vi "AccueilAdministrateur.vi"() -> ()   [LabVIEW 2015]
uses:
  Queues and Variants 8.2/Queue Element.ctl
  Queues and Variants 8.2/Data Type.ctl
  <vilib>/httpClient/LabVIEWHTTPClient.lvlib
panel:
  in  "OK Button 8":bool
  out "Boolean Out":bool
  out "String Out":string
  out "Double Precision Out":dbl
  in  "OK Button 7":bool
  in  "OK Button 6":bool
  in  "OK Button 5":bool
  in  "OK Button 4":bool
  in  "OK Button 3":bool
  in  "OK Button 2":bool
  in  "OK Button":bool
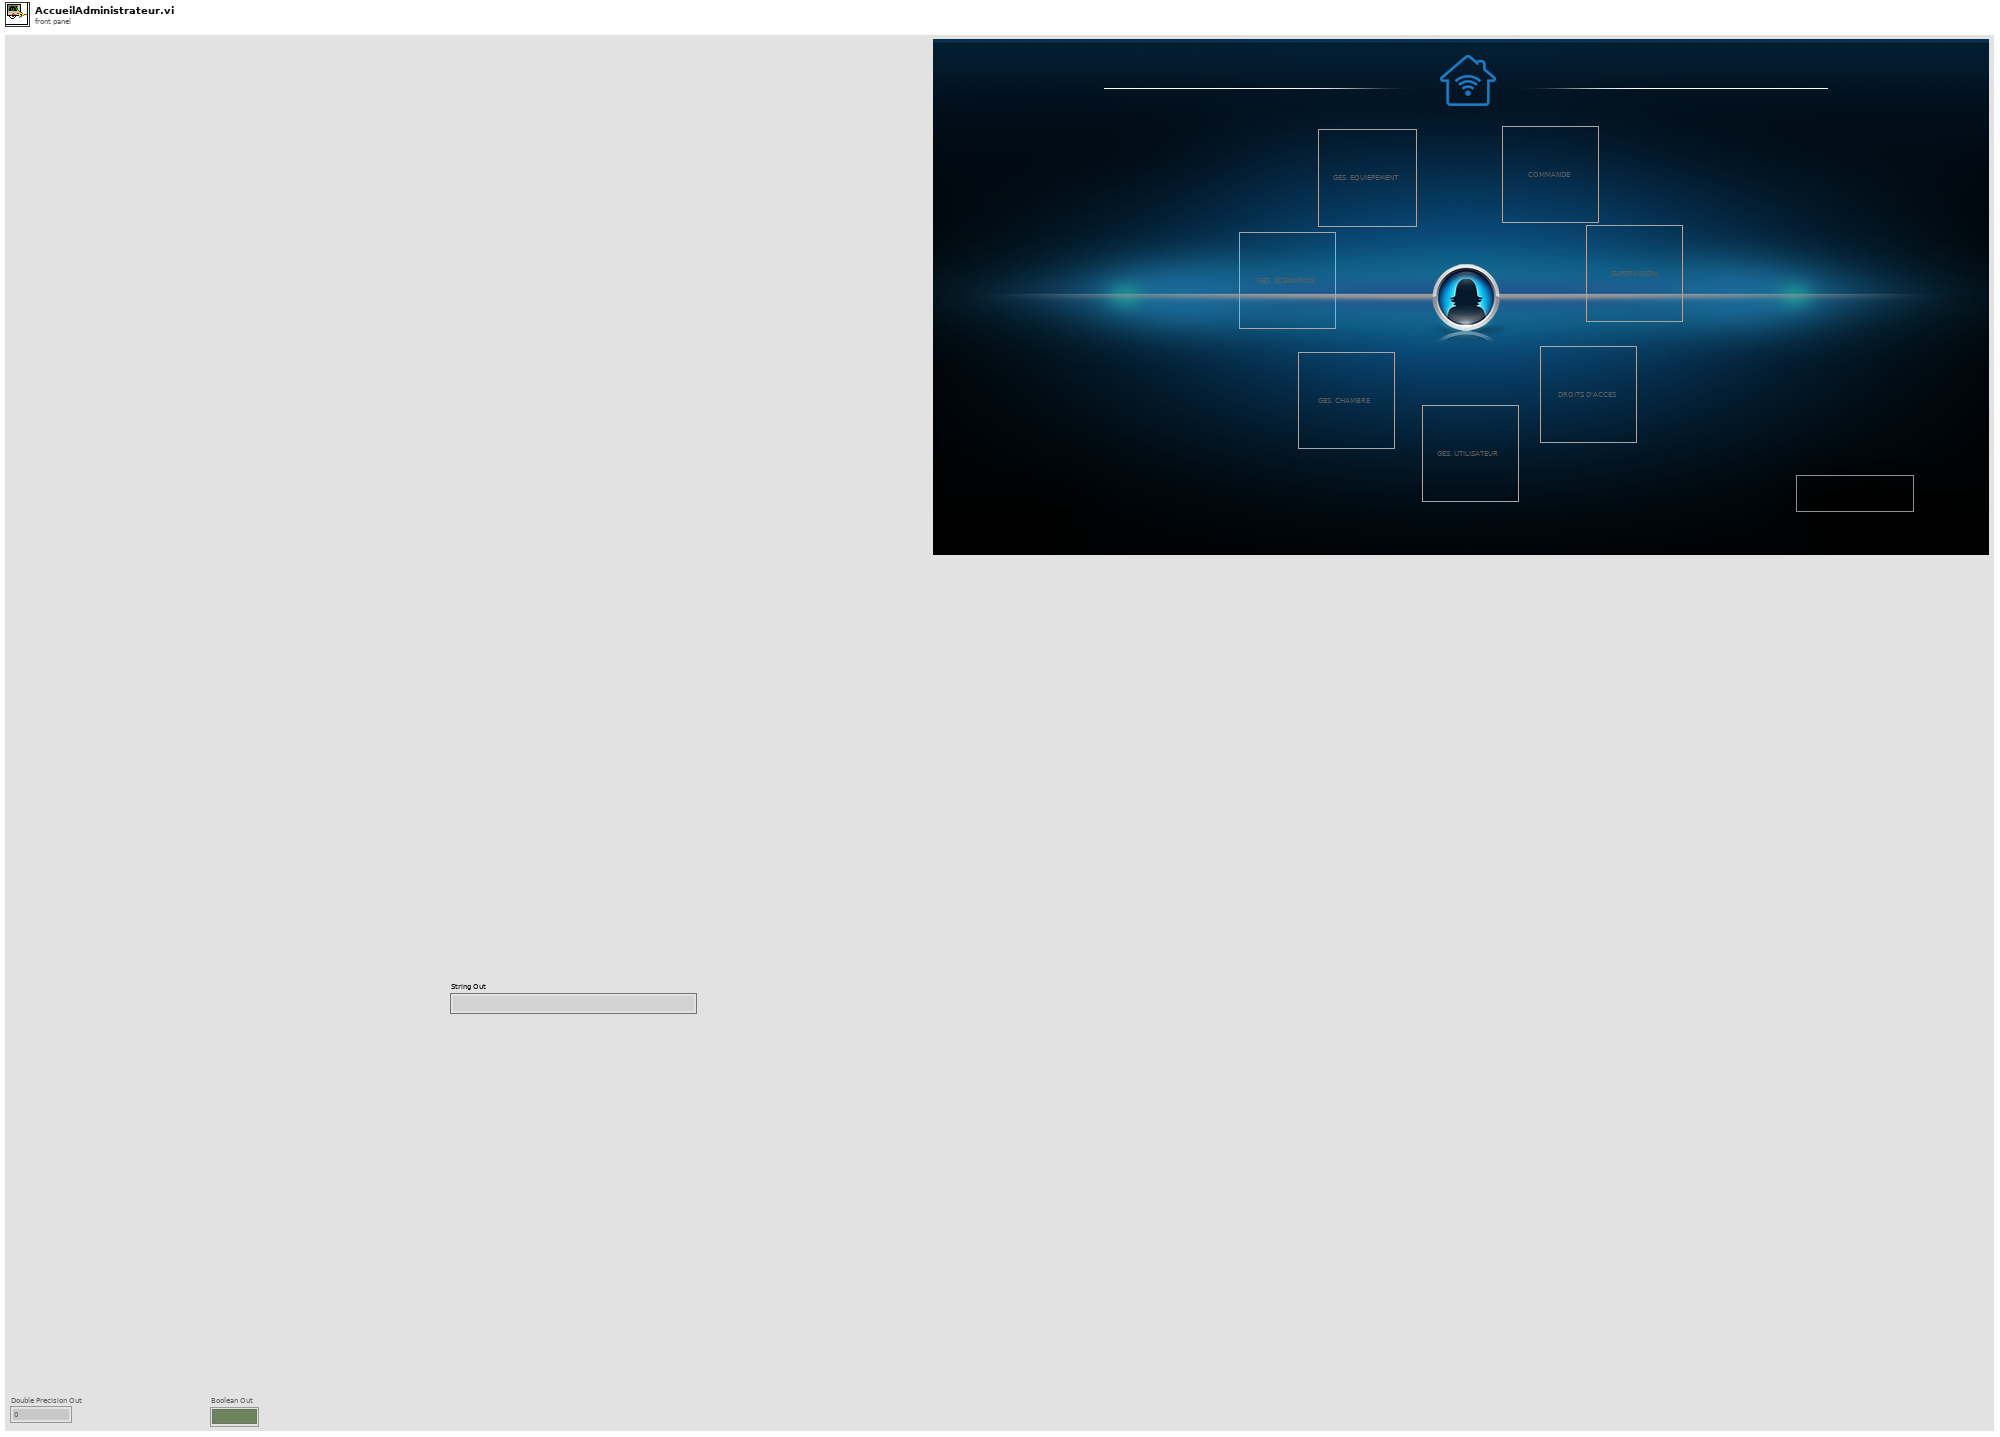
[diagram p1: front panel]
types:
  T1 = typedef "Queue Element.ctl" = cluster{"Data Type":T2, "Variant":variant}
  T2 = typedef "Data Type.ctl" = enum16{"Double Precision", "String", "Boolean"}
  T3 = enum32{"Invalid", "Standard", "Closed", "Hidden", "Minimized", "Maximized"}
  T4 = enum8{"Enabled", "Disabled", "Disabled and Grayed Out"}
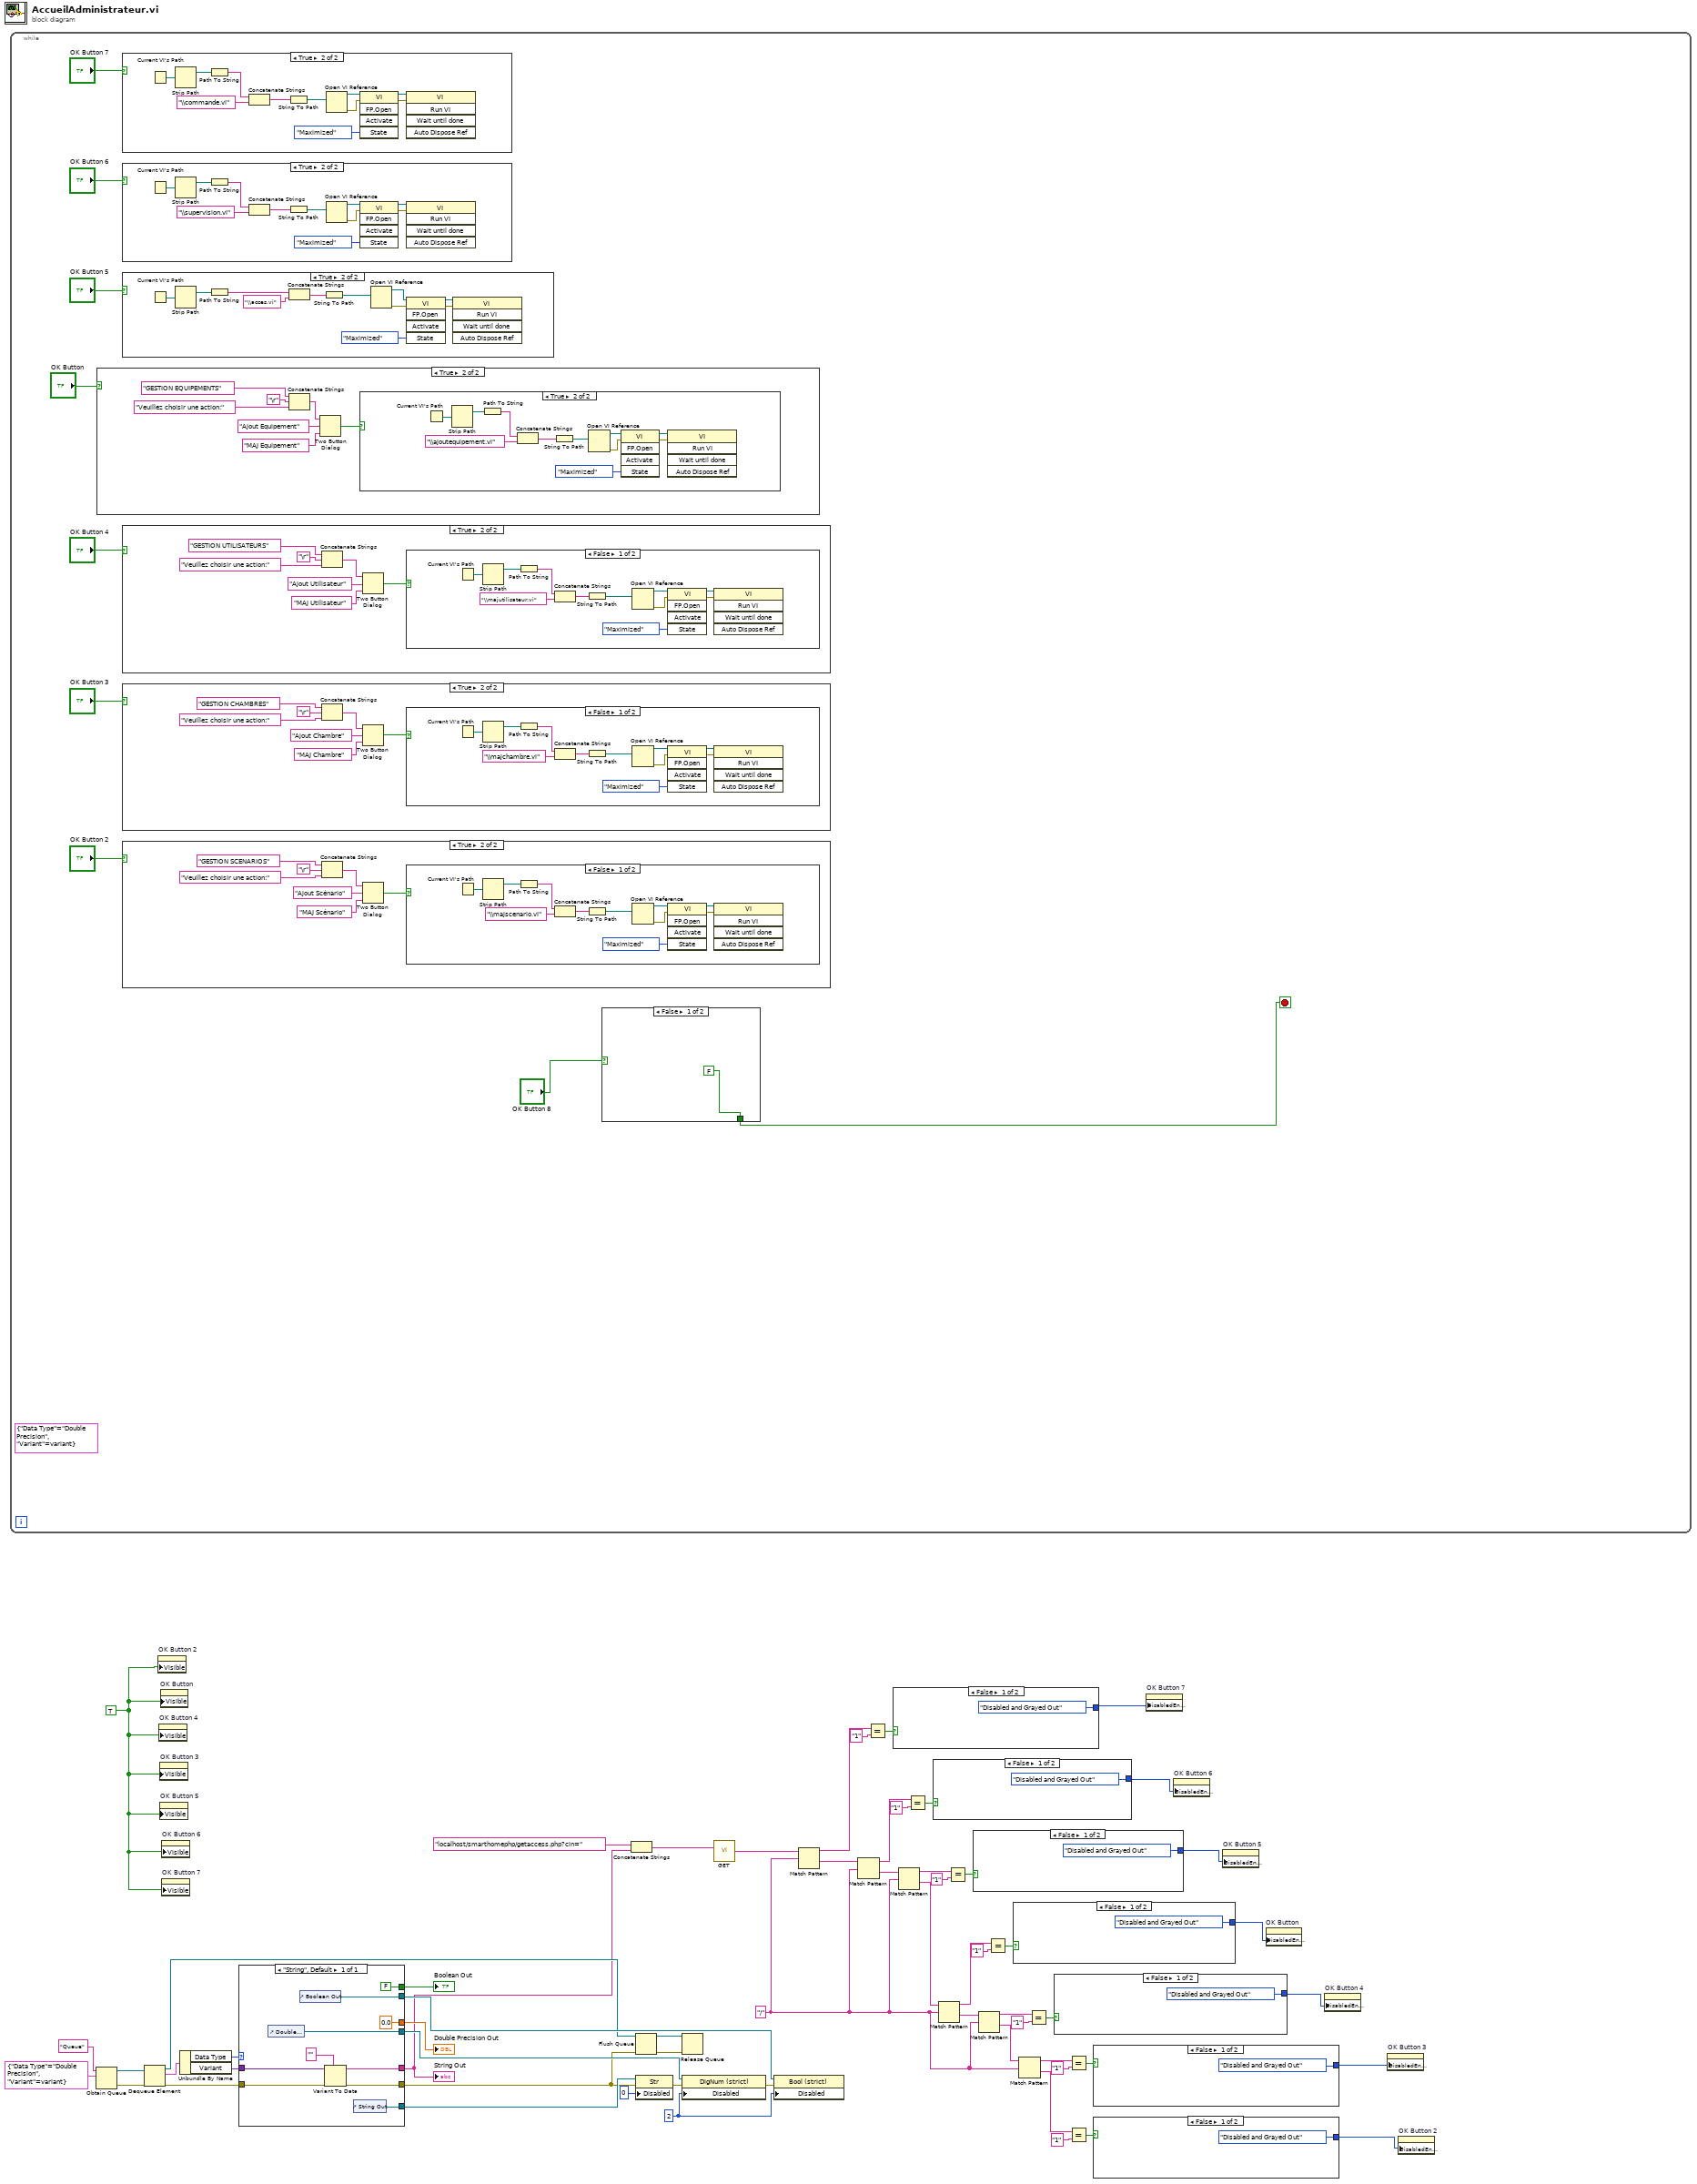
[diagram p0: block diagram]
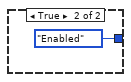
[diagram p2: hidden frame]
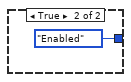
[diagram p3: hidden frame]
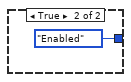
[diagram p4: hidden frame]
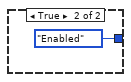
[diagram p5: hidden frame]
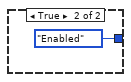
[diagram p6: hidden frame]
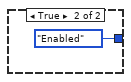
[diagram p7: hidden frame]
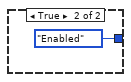
[diagram p8: hidden frame]
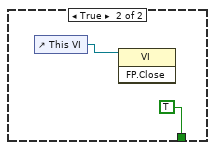
[diagram p9: hidden frame]
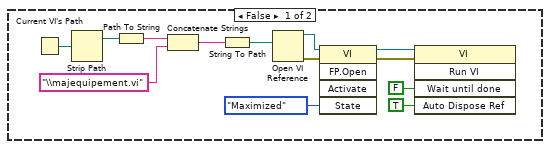
[diagram p14: hidden frame]
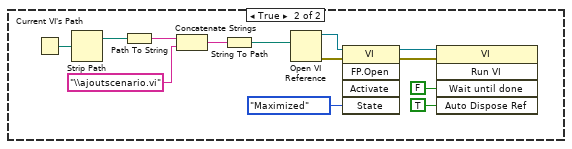
[diagram p16: hidden frame]
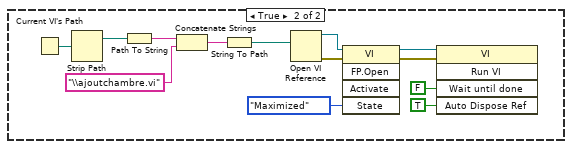
[diagram p18: hidden frame]
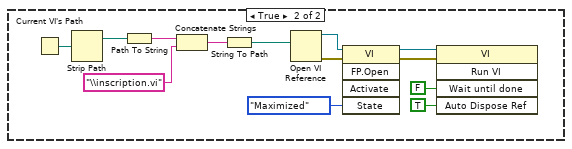
[diagram p20: hidden frame]
diagram:
  w26 = "/" ("regular expression")
  w44 = u8 2 ("Disabled")
  w53 = TRUE
  n1 = while {
    stop <- w61 stop-if-true
    (unwired) T1 {"Data Type"=enum."Double Precision", "Variant"=variant} ("Queue Element")
    n2 = case shown="True" "OK Button" {
      frame False {
      }
      frame True {
        n3 = Concatenate Strings("GESTION EQUIPEMENTS", "\r", "Veuillez choisir une action:" ("message")) -> (w109:string)
        n4 = Two Button Dialog(message=w109, 1:"MAJ Equipement" ("F button name (\"Cancel\")"), 2:"Ajout Equipement" ("T button name (\"OK\")")) -> (T button?=w106:bool)
        n5 = case shown="True" w106 {
          frame False {
            n6 = Current VI's Path() -> (path=w125:path)
            n7 = Strip Path(path=w125) -> (stripped path=w124:path)  [unwired: 1 out]
            n8 = Path To String(path=w124) -> (string=w123:string)
            n9 = Concatenate Strings(w123, "\\majequipement.vi") -> (w121:string)
            n10 = String To Path(string=w121) -> (path=w120:path)
            n11 = Open VI Reference(vi path=w120) -> (vi reference=w119:refnum<vi>, error out=w118:errorcluster)  [unwired: 5 in]
            n12 = invoke class="VI" method="FP.Open"(reference=w119, error in=w118, "State"=T3."Maximized") -> (reference out=w117:refnum<vi>, error out=w116:errorcluster)  [unwired: 2 in, 3 out]
            n13 = invoke class="VI" method="Run VI"(reference=w117, error in=w116, "Wait until done"=FALSE ("Wait Until Done"), "Auto Dispose Ref"=TRUE ("Auto Dispose Reference")) -> ()  [unwired: 1 in, 5 out]
          }
          frame True {
            n14 = Current VI's Path() -> (path=w136:path)
            n15 = Strip Path(path=w136) -> (stripped path=w135:path)  [unwired: 1 out]
            n16 = Path To String(path=w135) -> (string=w134:string)
            n17 = Concatenate Strings(w134, "\\ajoutequipement.vi") -> (w132:string)
            n18 = String To Path(string=w132) -> (path=w131:path)
            n19 = Open VI Reference(vi path=w131) -> (vi reference=w130:refnum<vi>, error out=w129:errorcluster)  [unwired: 5 in]
            n20 = invoke class="VI" method="FP.Open"(reference=w130, error in=w129, "State"=T3."Maximized") -> (reference out=w128:refnum<vi>, error out=w127:errorcluster)  [unwired: 2 in, 3 out]
            n21 = invoke class="VI" method="Run VI"(reference=w128, error in=w127) -> ()  [unwired: 3 in, 5 out]
          }
        }
      }
    }
    n22 = case shown="True" "OK Button 7" {
      frame False {
      }
      frame True {
        n23 = Current VI's Path() -> (path=w105:path)
        n24 = Strip Path(path=w105) -> (stripped path=w104:path)  [unwired: 1 out]
        n25 = Path To String(path=w104) -> (string=w103:string)
        n26 = Concatenate Strings(w103, "\\commande.vi") -> (w101:string)
        n27 = String To Path(string=w101) -> (path=w100:path)
        n28 = Open VI Reference(vi path=w100) -> (vi reference=w99:refnum<vi>, error out=w98:errorcluster)  [unwired: 5 in]
        n29 = invoke class="VI" method="FP.Open"(reference=w99, error in=w98, "State"=T3."Maximized") -> (reference out=w97:refnum<vi>, error out=w96:errorcluster)  [unwired: 2 in, 3 out]
        n30 = invoke class="VI" method="Run VI"(reference=w97, error in=w96) -> ()  [unwired: 3 in, 5 out]
      }
    }
    n31 = case shown="True" "OK Button 6" {
      frame False {
      }
      frame True {
        n32 = Current VI's Path() -> (path=w94:path)
        n33 = Strip Path(path=w94) -> (stripped path=w93:path)  [unwired: 1 out]
        n34 = Path To String(path=w93) -> (string=w92:string)
        n35 = Concatenate Strings(w92, "\\supervision.vi") -> (w90:string)
        n36 = String To Path(string=w90) -> (path=w89:path)
        n37 = Open VI Reference(vi path=w89) -> (vi reference=w88:refnum<vi>, error out=w87:errorcluster)  [unwired: 5 in]
        n38 = invoke class="VI" method="FP.Open"(reference=w88, error in=w87, "State"=T3."Maximized") -> (reference out=w86:refnum<vi>, error out=w85:errorcluster)  [unwired: 2 in, 3 out]
        n39 = invoke class="VI" method="Run VI"(reference=w86, error in=w85) -> ()  [unwired: 3 in, 5 out]
      }
    }
    n40 = case shown="True" "OK Button 5" {
      frame False {
      }
      frame True {
        n41 = Current VI's Path() -> (path=w83:path)
        n42 = Strip Path(path=w83) -> (stripped path=w82:path)  [unwired: 1 out]
        n43 = Path To String(path=w82) -> (string=w81:string)
        n44 = Concatenate Strings(w81, "\\acces.vi") -> (w79:string)
        n45 = String To Path(string=w79) -> (path=w78:path)
        n46 = Open VI Reference(vi path=w78) -> (vi reference=w77:refnum<vi>, error out=w76:errorcluster)  [unwired: 5 in]
        n47 = invoke class="VI" method="FP.Open"(reference=w77, error in=w76, "State"=T3."Maximized") -> (reference out=w75:refnum<vi>, error out=w74:errorcluster)  [unwired: 2 in, 3 out]
        n48 = invoke class="VI" method="Run VI"(reference=w75, error in=w74) -> ()  [unwired: 3 in, 5 out]
      }
    }
    n49 = case shown="True" "OK Button 4" {
      frame False {
      }
      frame True {
        n50 = Concatenate Strings("GESTION UTILISATEURS", "\r", "Veuillez choisir une action:" ("message")) -> (w202:string)
        n51 = Two Button Dialog(message=w202, 1:"MAJ Utilisateur" ("F button name (\"Cancel\")"), 2:"Ajout Utilisateur" ("T button name (\"OK\")")) -> (T button?=w199:bool)
        n52 = case shown="False" w199 {
          frame False {
            n53 = Current VI's Path() -> (path=w216:path)
            n54 = Strip Path(path=w216) -> (stripped path=w215:path)  [unwired: 1 out]
            n55 = Path To String(path=w215) -> (string=w214:string)
            n56 = Concatenate Strings(w214, "\\majutilisateur.vi") -> (w212:string)
            n57 = String To Path(string=w212) -> (path=w211:path)
            n58 = Open VI Reference(vi path=w211) -> (vi reference=w210:refnum<vi>, error out=w209:errorcluster)  [unwired: 5 in]
            n59 = invoke class="VI" method="FP.Open"(reference=w210, error in=w209, "State"=T3."Maximized") -> (reference out=w208:refnum<vi>, error out=w207:errorcluster)  [unwired: 2 in, 3 out]
            n60 = invoke class="VI" method="Run VI"(reference=w208, error in=w207) -> ()  [unwired: 3 in, 5 out]
          }
          frame True {
            n61 = Current VI's Path() -> (path=w229:path)
            n62 = Strip Path(path=w229) -> (stripped path=w228:path)  [unwired: 1 out]
            n63 = Path To String(path=w228) -> (string=w227:string)
            n64 = Concatenate Strings(w227, "\\inscription.vi") -> (w225:string)
            n65 = String To Path(string=w225) -> (path=w224:path)
            n66 = Open VI Reference(vi path=w224) -> (vi reference=w223:refnum<vi>, error out=w222:errorcluster)  [unwired: 5 in]
            n67 = invoke class="VI" method="FP.Open"(reference=w223, error in=w222, "State"=T3."Maximized") -> (reference out=w221:refnum<vi>, error out=w220:errorcluster)  [unwired: 2 in, 3 out]
            n68 = invoke class="VI" method="Run VI"(reference=w221, error in=w220, "Wait until done"=FALSE ("Wait Until Done"), "Auto Dispose Ref"=TRUE ("Auto Dispose Reference")) -> ()  [unwired: 1 in, 5 out]
          }
        }
      }
    }
    n69 = case shown="True" "OK Button 3" {
      frame False {
      }
      frame True {
        n70 = Concatenate Strings("GESTION CHAMBRES", "\r", "Veuillez choisir une action:" ("message")) -> (w171:string)
        n71 = Two Button Dialog(message=w171, 1:"MAJ Chambre" ("F button name (\"Cancel\")"), 2:"Ajout Chambre" ("T button name (\"OK\")")) -> (T button?=w168:bool)
        n72 = case shown="False" w168 {
          frame False {
            n73 = Current VI's Path() -> (path=w185:path)
            n74 = Strip Path(path=w185) -> (stripped path=w184:path)  [unwired: 1 out]
            n75 = Path To String(path=w184) -> (string=w183:string)
            n76 = Concatenate Strings(w183, "\\majchambre.vi") -> (w181:string)
            n77 = String To Path(string=w181) -> (path=w180:path)
            n78 = Open VI Reference(vi path=w180) -> (vi reference=w179:refnum<vi>, error out=w178:errorcluster)  [unwired: 5 in]
            n79 = invoke class="VI" method="FP.Open"(reference=w179, error in=w178, "State"=T3."Maximized") -> (reference out=w177:refnum<vi>, error out=w176:errorcluster)  [unwired: 2 in, 3 out]
            n80 = invoke class="VI" method="Run VI"(reference=w177, error in=w176) -> ()  [unwired: 3 in, 5 out]
          }
          frame True {
            n81 = Current VI's Path() -> (path=w198:path)
            n82 = Strip Path(path=w198) -> (stripped path=w197:path)  [unwired: 1 out]
            n83 = Path To String(path=w197) -> (string=w196:string)
            n84 = Concatenate Strings(w196, "\\ajoutchambre.vi") -> (w194:string)
            n85 = String To Path(string=w194) -> (path=w193:path)
            n86 = Open VI Reference(vi path=w193) -> (vi reference=w192:refnum<vi>, error out=w191:errorcluster)  [unwired: 5 in]
            n87 = invoke class="VI" method="FP.Open"(reference=w192, error in=w191, "State"=T3."Maximized") -> (reference out=w190:refnum<vi>, error out=w189:errorcluster)  [unwired: 2 in, 3 out]
            n88 = invoke class="VI" method="Run VI"(reference=w190, error in=w189, "Wait until done"=FALSE ("Wait Until Done"), "Auto Dispose Ref"=TRUE ("Auto Dispose Reference")) -> ()  [unwired: 1 in, 5 out]
          }
        }
      }
    }
    n89 = case shown="True" "OK Button 2" {
      frame False {
      }
      frame True {
        n90 = Concatenate Strings("GESTION SCENARIOS", "\r", "Veuillez choisir une action:" ("message")) -> (w140:string)
        n91 = Two Button Dialog(message=w140, 1:"MAJ Scénario" ("F button name (\"Cancel\")"), 2:"Ajout Scénario" ("T button name (\"OK\")")) -> (T button?=w137:bool)
        n92 = case shown="False" w137 {
          frame False {
            n93 = Current VI's Path() -> (path=w154:path)
            n94 = Strip Path(path=w154) -> (stripped path=w153:path)  [unwired: 1 out]
            n95 = Path To String(path=w153) -> (string=w152:string)
            n96 = Concatenate Strings(w152, "\\majscenario.vi") -> (w150:string)
            n97 = String To Path(string=w150) -> (path=w149:path)
            n98 = Open VI Reference(vi path=w149) -> (vi reference=w148:refnum<vi>, error out=w147:errorcluster)  [unwired: 5 in]
            n99 = invoke class="VI" method="FP.Open"(reference=w148, error in=w147, "State"=T3."Maximized") -> (reference out=w146:refnum<vi>, error out=w145:errorcluster)  [unwired: 2 in, 3 out]
            n100 = invoke class="VI" method="Run VI"(reference=w146, error in=w145) -> ()  [unwired: 3 in, 5 out]
          }
          frame True {
            n101 = Current VI's Path() -> (path=w167:path)
            n102 = Strip Path(path=w167) -> (stripped path=w166:path)  [unwired: 1 out]
            n103 = Path To String(path=w166) -> (string=w165:string)
            n104 = Concatenate Strings(w165, "\\ajoutscenario.vi") -> (w163:string)
            n105 = String To Path(string=w163) -> (path=w162:path)
            n106 = Open VI Reference(vi path=w162) -> (vi reference=w161:refnum<vi>, error out=w160:errorcluster)  [unwired: 5 in]
            n107 = invoke class="VI" method="FP.Open"(reference=w161, error in=w160, "State"=T3."Maximized") -> (reference out=w159:refnum<vi>, error out=w158:errorcluster)  [unwired: 2 in, 3 out]
            n108 = invoke class="VI" method="Run VI"(reference=w159, error in=w158, "Wait until done"=FALSE ("Wait Until Done"), "Auto Dispose Ref"=TRUE ("Auto Dispose Reference")) -> ()  [unwired: 1 in, 5 out]
          }
        }
      }
    }
    n109 = case shown="False" "OK Button 8" {
      tunnel: [FALSE TRUE] -> w61
      frame False {
      }
      frame True {
        n110 = control-ref of="This VI"() -> (w72:refnum<vi>)
        n111 = invoke class="VI" method="FP.Close"(reference=w72) -> ()  [unwired: 2 in, 3 out]
      }
    }
  }
  n112 = Obtain Queue(name (unnamed)="Queue", element data type=T1 {"Data Type"=enum."Double Precision", "Variant"=variant} ("Queue Element")) -> (queue out=w2:refnum<queue>, error out=w1:errorcluster)  [unwired: 3 in, 1 out]
  n113 = Dequeue Element(queue=w2, error in (no error)=w1) -> (queue out=w40:refnum<queue>, element=w41:T1, error out=w51:errorcluster)  [unwired: 1 in, 1 out]
  n114 = property on="OK Button 2" class="Bool"("Visible"=w53) -> ()  [unwired: 2 in, 2 out]
  n115 = property on="OK Button 4" class="Bool"("Visible"=w53) -> ()  [unwired: 2 in, 2 out]
  n116 = property on="OK Button 3" class="Bool"("Visible"=w53) -> ()  [unwired: 2 in, 2 out]
  n117 = property on="OK Button 5" class="Bool"("Visible"=w53) -> ()  [unwired: 2 in, 2 out]
  n118 = property on="OK Button" class="Bool"("Visible"=w53) -> ()  [unwired: 2 in, 2 out]
  n119 = property on="OK Button 6" class="Bool"("Visible"=w53) -> ()  [unwired: 2 in, 2 out]
  n120 = property on="OK Button 7" class="Bool"("Visible"=w53) -> ()  [unwired: 2 in, 2 out]
  n121 = Unbundle By Name(w41) -> ("Data Type"=w36:T2, "Variant"=w52:variant)
  n122 = case shown="\"String\", Default" w36 {
    tunnel: w52 -> [w230]
    tunnel: w51 -> [w238]
    tunnel: [0.0] -> w43
    tunnel: [w237] -> w34
    tunnel: [FALSE] -> w42
    tunnel: [w234] -> w50
    tunnel: [w233] -> w48
    tunnel: [w232] -> w47
    tunnel: [w231] -> w37
    frame "String", Default {
      n123 = control-ref of="Double Precision Out"() -> (w233:refnum<vi>)
      n124 = control-ref of="Boolean Out"() -> (w232:refnum<vi>)
      n125 = Variant To Data(error in=w238, type="", Variant=w230) -> (data=w237:string, error out=w231:errorcluster)
      n126 = control-ref of="String Out"() -> (w234:refnum<vi>)
    }
  }
  "Double Precision Out" <- w43
  "String Out" <- w34
  "Boolean Out" <- w42
  n127 = Concatenate Strings("localhost/smarthomephp/getaccess.php?cin=", w34) -> (w33:string)
  n128 = Flush Queue(queue=w40, error in (no error)=w37) -> (queue out=w39:refnum<queue>, error out=w38:errorcluster)  [unwired: 1 out]
  n129 = property class="Str"(reference=w50, error in=w37, "Disabled"=u8 0) -> (error out=w46:errorcluster)  [unwired: 1 out]
  n130 = Release Queue(queue=w39, error in (no error)=w38) -> ()  [unwired: 4 out]
  n131 = property class="DigNum (strict)"(reference=w48, error in=w46, "Disabled"=w44) -> (error out=w45:errorcluster)  [unwired: 1 out]
  n132 = call <vilib>:"GET.vi"("url"=w33) -> ("body"=w32:string)  [unwired: 11 in, 3 out]
  n133 = property class="Bool (strict)"(reference=w47, error in=w45, "Disabled"=w44) -> ()  [unwired: 2 out]
  n134 = Match Pattern(string=w32, regular expression=w26) -> (before substring=w19:string, after substring=w31:string)  [unwired: 1 in, 2 out]
  n135 = Match Pattern(string=w31, regular expression=w26) -> (before substring=w20:string, after substring=w30:string)  [unwired: 1 in, 2 out]
  n136 = Equal?(x=w19, y="1") -> (x = y?=w18:bool)
  n137 = case shown="False" w18 {
    tunnel: [T4."Disabled and Grayed Out" ("Disabled") T4."Enabled" ("Disabled")] -> w54
    frame False {
    }
    frame True {
    }
  }
  n138 = Match Pattern(string=w30, regular expression=w26) -> (before substring=w21:string, after substring=w29:string)  [unwired: 1 in, 2 out]
  n139 = Equal?(x=w20, y="1") -> (x = y?=w17:bool)
  n140 = case shown="False" w17 {
    tunnel: [T4."Disabled and Grayed Out" ("Disabled") T4."Enabled" ("Disabled")] -> w55
    frame False {
    }
    frame True {
    }
  }
  n141 = Match Pattern(string=w29, regular expression=w26) -> (before substring=w14:string, after substring=w27:string)  [unwired: 1 in, 2 out]
  n142 = Equal?(x=w21, y="1") -> (x = y?=w16:bool)
  n143 = case shown="False" w16 {
    tunnel: [T4."Disabled and Grayed Out" ("Disabled") T4."Enabled" ("Disabled")] -> w56
    frame False {
    }
    frame True {
    }
  }
  n144 = Match Pattern(string=w27, regular expression=w26) -> (before substring=w13:string, after substring=w28:string)  [unwired: 1 in, 2 out]
  n145 = Equal?(x=w14, y="1") -> (x = y?=w15:bool)
  n146 = case shown="False" w15 {
    tunnel: [T4."Disabled and Grayed Out" ("Disabled") T4."Enabled" ("Disabled")] -> w57
    frame False {
    }
    frame True {
    }
  }
  n147 = Match Pattern(string=w28, regular expression=w26) -> (before substring=w10:string, after substring=w5:string)  [unwired: 1 in, 2 out]
  n148 = Equal?(x=w13, y="1") -> (x = y?=w12:bool)
  n149 = case shown="False" w12 {
    tunnel: [T4."Disabled and Grayed Out" ("Disabled") T4."Enabled" ("Disabled")] -> w58
    frame False {
    }
    frame True {
    }
  }
  n150 = Equal?(x=w10, y="1") -> (x = y?=w8:bool)
  n151 = Equal?(x=w5, y="1") -> (x = y?=w7:bool)
  n152 = case shown="False" w8 {
    tunnel: [T4."Disabled and Grayed Out" ("Disabled") T4."Enabled" ("Disabled")] -> w59
    frame False {
    }
    frame True {
    }
  }
  n153 = case shown="False" w7 {
    tunnel: [T4."Disabled and Grayed Out" ("Disabled") T4."Enabled" ("Disabled")] -> w60
    frame False {
    }
    frame True {
    }
  }
  n154 = property on="OK Button 7" class="Bool"("DisabledEnum"=w54) -> ()  [unwired: 2 in, 2 out]
  n155 = property on="OK Button 6" class="Bool"("DisabledEnum"=w55) -> ()  [unwired: 2 in, 2 out]
  n156 = property on="OK Button 5" class="Bool"("DisabledEnum"=w56) -> ()  [unwired: 2 in, 2 out]
  n157 = property on="OK Button" class="Bool"("DisabledEnum"=w57) -> ()  [unwired: 2 in, 2 out]
  n158 = property on="OK Button 4" class="Bool"("DisabledEnum"=w58) -> ()  [unwired: 2 in, 2 out]
  n159 = property on="OK Button 3" class="Bool"("DisabledEnum"=w59) -> ()  [unwired: 2 in, 2 out]
  n160 = property on="OK Button 2" class="Bool"("DisabledEnum"=w60) -> ()  [unwired: 2 in, 2 out]
